vi "THE EXECUTION TIME CHECK.vi"() -> ()   [LabVIEW 2015]
panel:
  out "THE RESULT":string
  out "Y":dbl
  in  "X":dbl
  out "EXECUTION TIME":dbl
  out "EXECUTION TIME":dbl
  out "Y":dbl
  in  "X":dbl
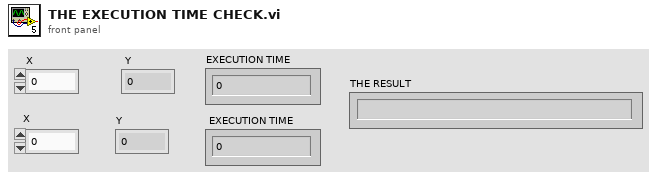
[diagram p1: front panel]
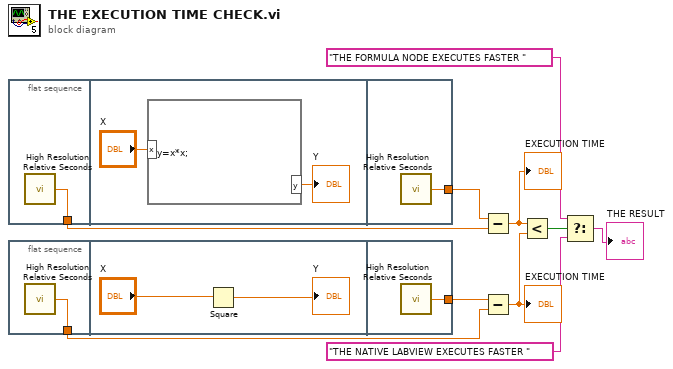
[diagram p0: block diagram]
diagram:
  n1 = flat-sequence {
    tunnel: [w11] -> w10
    tunnel: [w14] -> w9
    frame #0 {
      n2 = call <vilib>:"High Resolution Relative Seconds.vi"() -> ("relative seconds"=w11:dbl)
    }
    frame #1 {
      n3 = formula code="y=x*x;"("x"="X") -> ("y"=→"Y":dbl)
    }
    frame #2 {
      n4 = call <vilib>:"High Resolution Relative Seconds.vi"() -> ("relative seconds"=w14:dbl)
    }
  }
  n5 = flat-sequence {
    tunnel: [w15] -> w8
    tunnel: [w18] -> w7
    frame #0 {
      n6 = call <vilib>:"High Resolution Relative Seconds.vi"() -> ("relative seconds"=w15:dbl)
    }
    frame #1 {
      n7 = Square(x="X") -> (x^2=→"Y":dbl)
    }
    frame #2 {
      n8 = call <vilib>:"High Resolution Relative Seconds.vi"() -> ("relative seconds"=w18:dbl)
    }
  }
  n9 = Subtract(x=w9, y=w10) -> (x-y=w6:dbl)
  "EXECUTION TIME" <- w6
  n10 = Subtract(x=w7, y=w8) -> (x-y=w5:dbl)
  "EXECUTION TIME" <- w5
  n11 = Less?(x=w6, y=w5) -> (x < y?=w4:bool)
  n12 = Select(t="THE FORMULA NODE EXECUTES FASTER ", s=w4, f="THE NATIVE LABVIEW EXECUTES FASTER ") -> (s? t:f=→"THE RESULT":string)
